vi "Get UID.vi"(8 "error in (no error)":errorcluster, 11 "LV Doc.lvclass":refnum<class "LV Doc.lvclass">) -> (0 "error out":errorcluster, 3 "LV Doc.lvclass":refnum<class "LV Doc.lvclass">)   [LabVIEW 2016, in "LV Doc.lvclass"]
uses:
  LV Doc.lvclass
  D:/MDI Project/source code/Document/Document.lvclass
  Document.lvclass/Document.ctl
  Document.lvclass
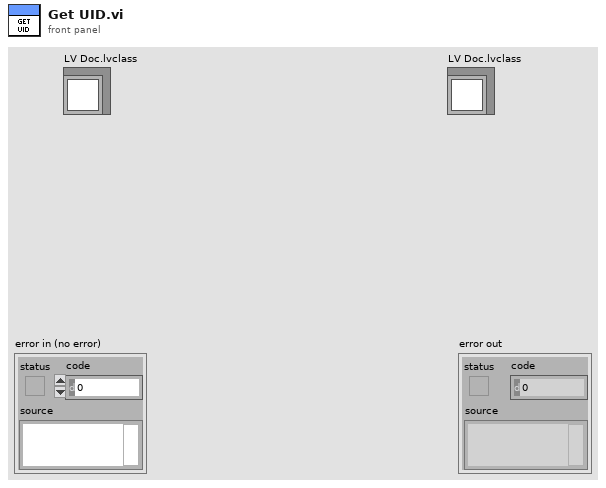
[diagram p1: front panel]
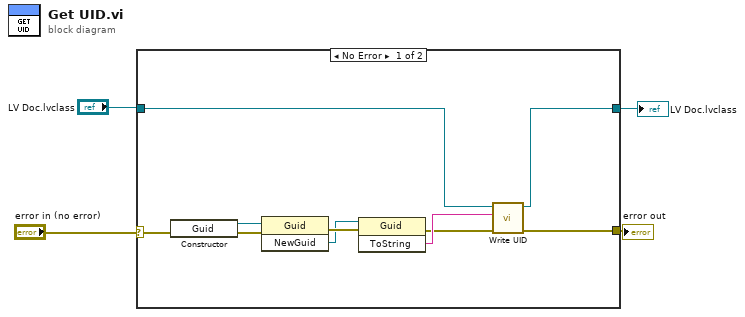
[diagram p0: block diagram]
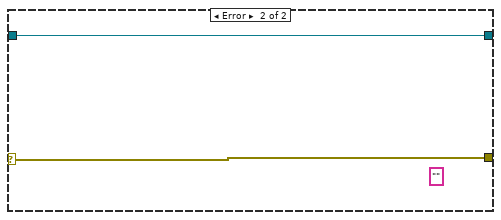
[diagram p2: hidden frame]
diagram:
  n1 = case shown="No Error" "error in (no error)" {
    selector: "error in (no error)" -> [w10 w16]
    tunnel: [w7 w16] -> w3
    tunnel: [w5 w15] -> w1
    tunnel: "LV Doc.lvclass" -> [w6 w15]
    frame No Error {
      n2 = constructor class="Guid"(error in=w10) -> (reference out=w11:refnum<k24>, error out=w12:errorcluster)  [unwired: 2 in, 1 out]
      n3 = invoke class="Guid" method="NewGuid"(reference=w11, error in=w12) -> (error out=w14:errorcluster, "NewGuid"=w13:refnum<k24>)  [unwired: 1 in, 1 out]
      n4 = invoke class="Guid" method="ToString"(reference=w13, error in=w14) -> (error out=w8:errorcluster, "ToString"=w9:string)  [unwired: 1 in, 1 out]
      n5 = call "Write UID.vi"("error in (no error)"=w8, "UID"=w9, "Document in"=w6) -> ("error out"=w7:errorcluster, "Document out"=w5:refnum<class "LV Doc.lvclass">)  [unwired: 7 in]
    }
    frame Error {
      (unwired) "" ("ToString")
    }
  }
  "error out" <- w3
  "LV Doc.lvclass" <- w1
